vi "Test Sequence.vi"(0 "FeedBack Channel":string[](array[string])=["fgdgfvcbc", "vnfhgjkn", "21354682"], 1 "Test Name":string, 2 "Steps":T1(array[cluster]), 3 "Load":refnum<vi>) -> (6 "Emergency":bool, 7 "Out":i32, 8 "Condition":bool)   [LabVIEW 2015]
uses:
  <vilib>/Utility/error.llb/whitespace.ctl
  Galobal variable_TI.vi
  Project Setup/Globle Variable/GR_Servo.vi
panel:
  out "Wait/Poll (ms)":u32
  out "Channels (Out)":i32[](array[numeric])
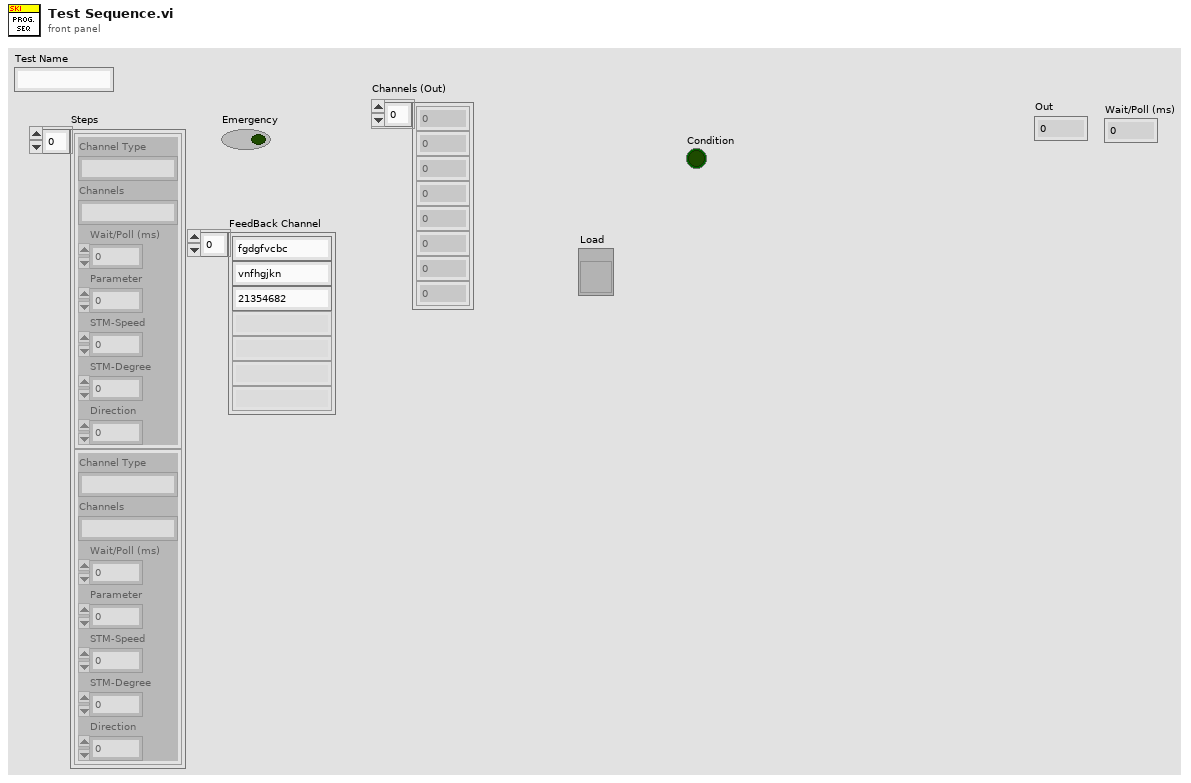
[diagram p1: front panel]
types:
  T1 = cluster{"Channel Type":string, "Channels":string, "Wait/Poll (ms)":u32, "Parameter":u8, "STM-Speed":i32, "STM-Degree":u32, "Direction":u8}[]
  T2 = cluster{"Emergency_1":bool, "Reset_2":bool, "Air Pressure_4":bool, "Safety Sensor_5":bool, "Safety Sensor_6":bool, "Barcode Rev rs_24":bool, "Clamp fwd rs_21":bool, "Servo Fault":bool, "Home _3":bool}
  T3 = cluster{"Start":bool, "Emergency ":bool, "Reset":bool, "Home":bool, "Safety":bool}
  T4 = typedef "whitespace.ctl" = u16
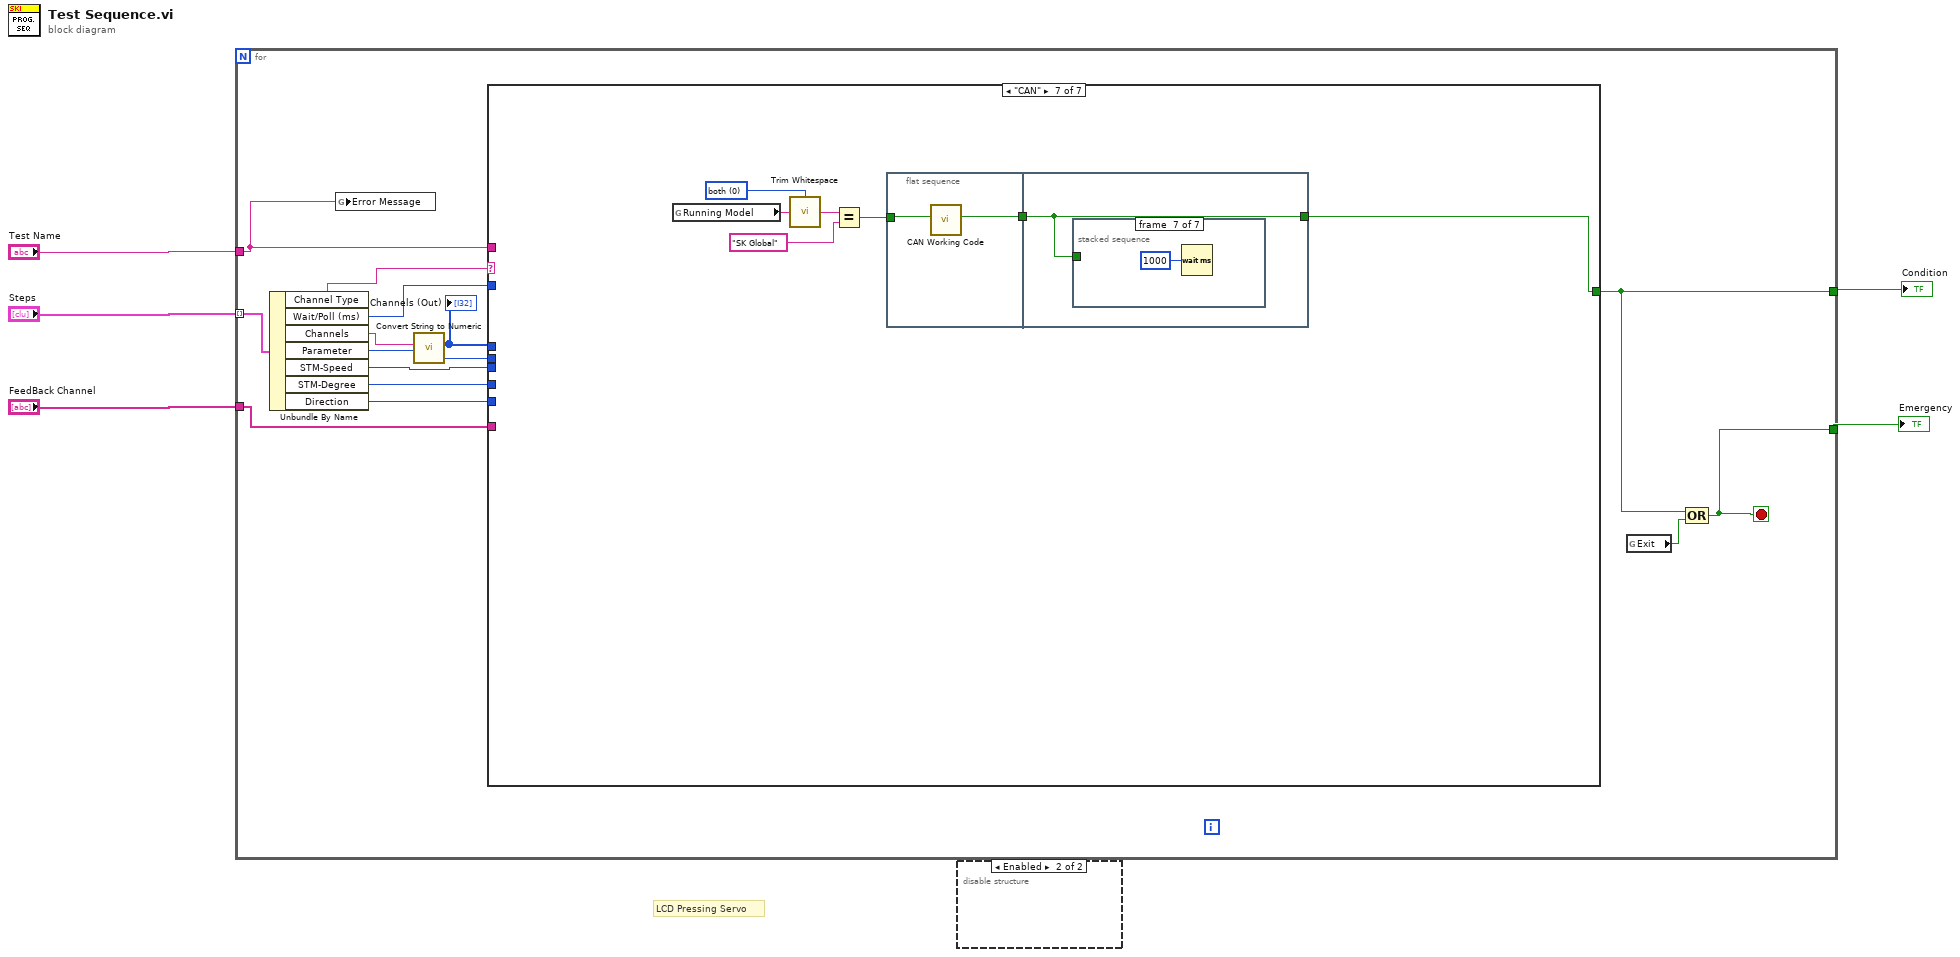
[diagram p0: block diagram]
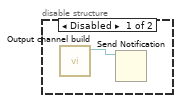
[diagram p2: hidden frame]
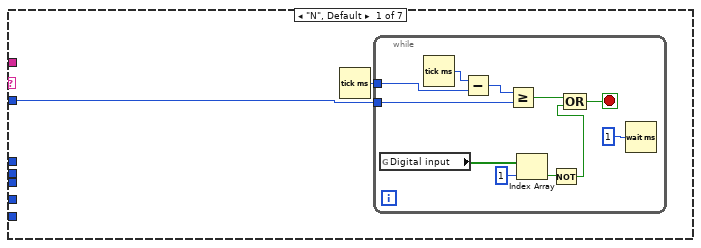
[diagram p3: hidden frame]
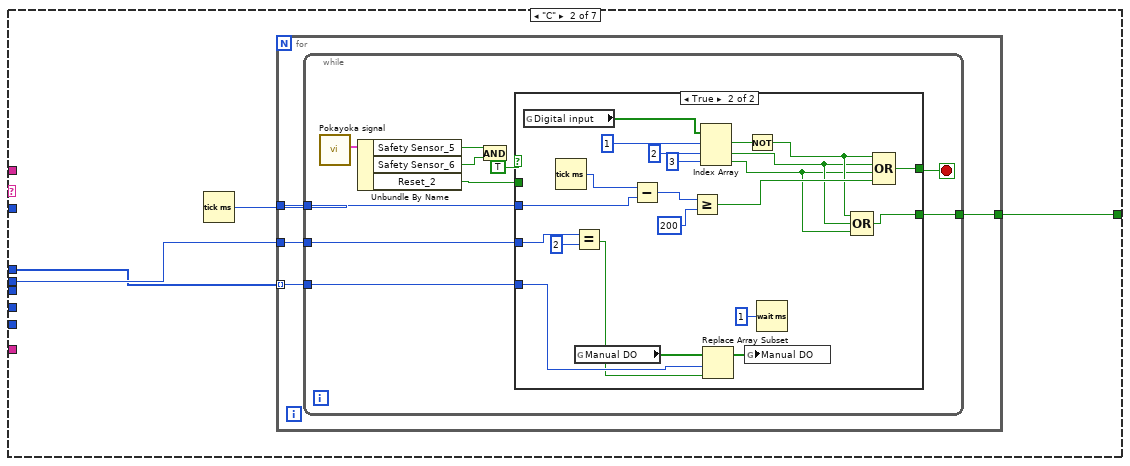
[diagram p4: hidden frame]
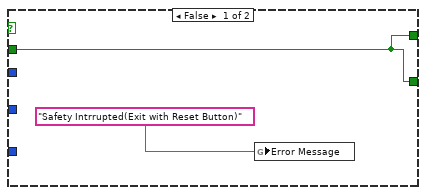
[diagram p5: hidden frame]
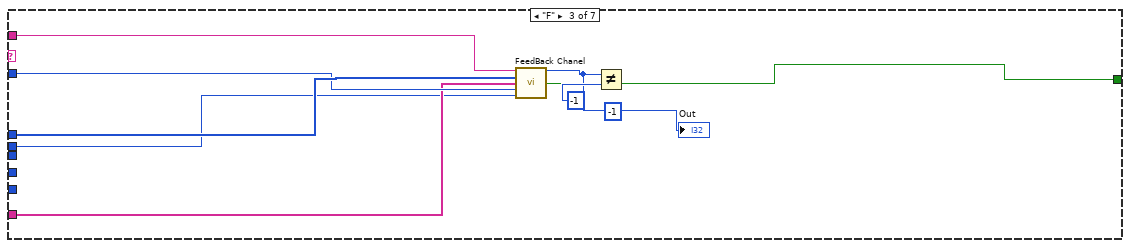
[diagram p6: hidden frame]
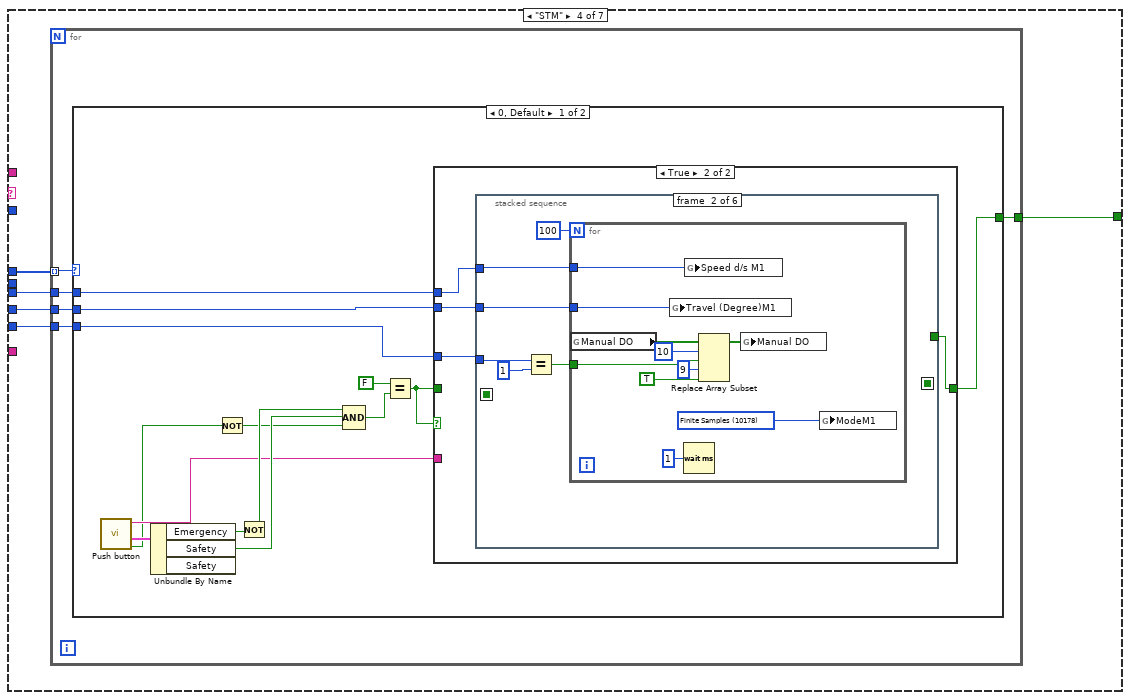
[diagram p7: hidden frame]
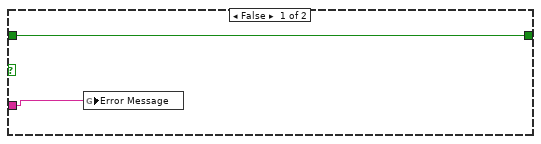
[diagram p8: hidden frame]
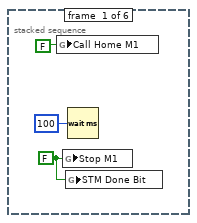
[diagram p9: hidden frame]
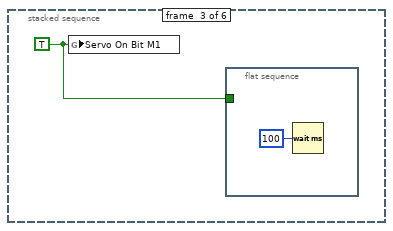
[diagram p10: hidden frame]
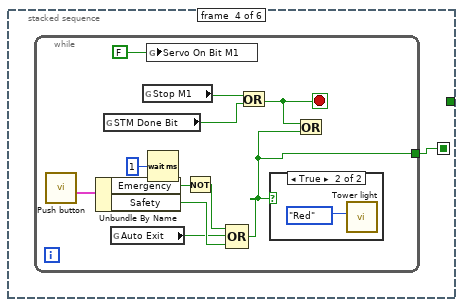
[diagram p11: hidden frame]
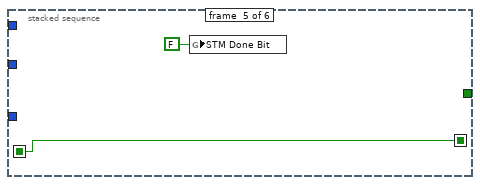
[diagram p13: hidden frame]
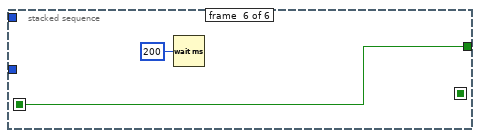
[diagram p14: hidden frame]
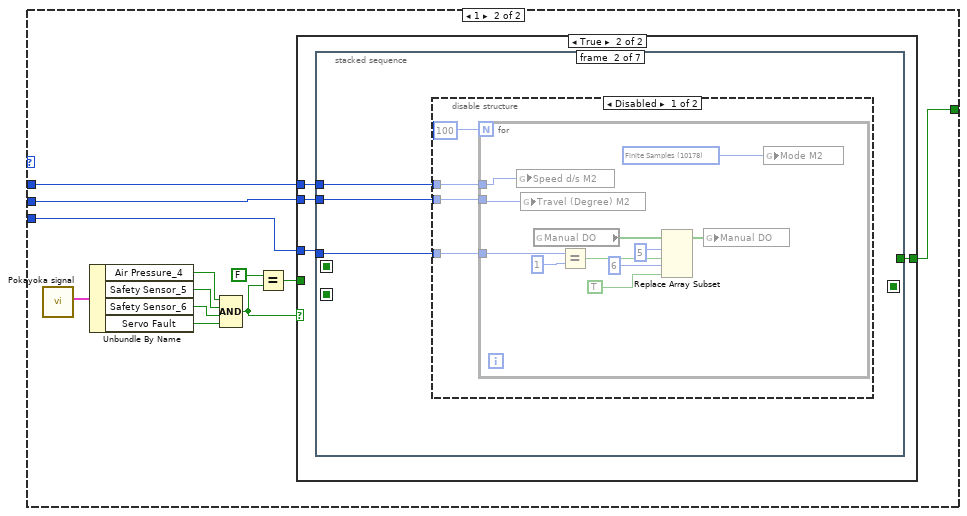
[diagram p15: hidden frame]
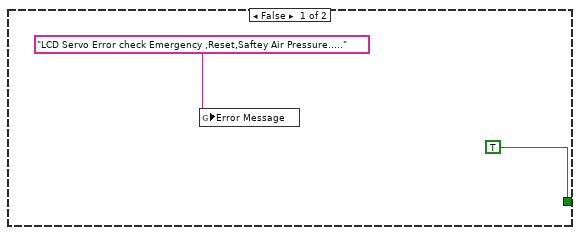
[diagram p16: hidden frame]
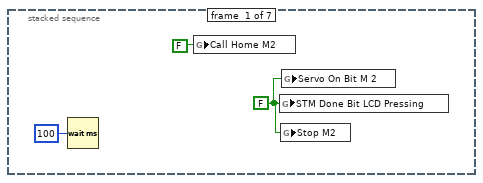
[diagram p17: hidden frame]
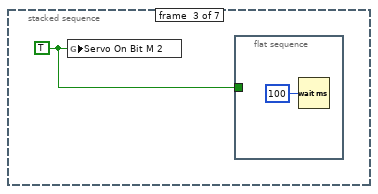
[diagram p19: hidden frame]
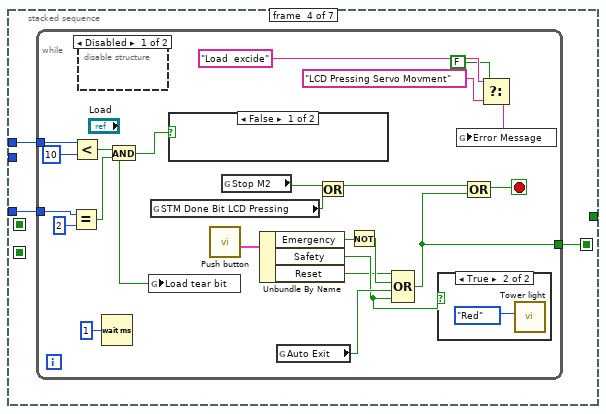
[diagram p20: hidden frame]
diagram:
  # "LCD Pressing Servo"
  n1 = for {
    tunnel: "Steps" -> [w19] mode=indexing
    tunnel: [w7] -> w5
    tunnel: "Test Name" -> [w6]
    tunnel: "FeedBack Channel" -> [w14]
    tunnel: [w12] -> w1
    stop <- w7 stop-if-true
    n2 = Unbundle By Name(w19) -> ("Channel Type"=w18:string, "Wait/Poll (ms)"=w17:u32, "Channels"=w16:string, "Parameter"=w8:u8, "STM-Speed"=w10:i32, "STM-Degree"=w9:u32, "Direction"=w11:u8)
    n3 = global write "GR_Servo.vi" "Error Message"(w6) -> ()
    n4 = call "Convert String to Numeric.vi"("Channels (A:B:C:D...) (In)"=w16) -> ("Channels (Out)"=w15:i32[])  [unwired: 9 in, 1 out]
    "Channels (Out)" <- w15
    n5 = case shown="\"CAN\"" w18 {
      tunnel: w17 -> [w20 _ w81 _ _ w273 _]
      tunnel: w15 -> [_ w34 w82 w87 w247 w274 _]
      tunnel: w11 -> [_ _ _ w86 _ _ _]
      tunnel: w6 -> [_ _ w80 _ _ _ _]
      tunnel: w14 -> [_ _ w79 _ _ _ _]
      tunnel: [_ w33 w75 w83 w245 w271 w318] -> w12
      tunnel: w10 -> [_ _ _ w85 _ _ _]
      tunnel: w9 -> [_ _ _ w84 _ _ _]
      tunnel: w8 -> [_ w36 w76 _ w246 w278 _]
      frame "N", Default {
        n6 = Tick Count (ms)() -> (millisecond timer value=w21:u32)
        n7 = while {
          tunnel: w21 -> [w31]
          tunnel: w20 -> [w26]
          stop <- w27 stop-if-true
          n8 = global read "Galobal variable_TI.vi" "Digital input"() -> (w25:bool[])
          n9 = Tick Count (ms)() -> (millisecond timer value=w32:u32)
          n10 = Subtract(x=w32, y=w31) -> (x-y=w30:u32)
          n11 = Greater Or Equal?(x=w30, y=w26) -> (x >= y?=w28:bool)
          n12 = Index Array(array=w25, index=1) -> (element=w23:bool)
          n13 = Not(x=w23) -> (.not. x?=w22:bool)
          n14 = Compound Arithmetic op=OR(w28, w22) -> (w27:bool)
          n15 = Wait (ms)(milliseconds to wait=u32 1) -> ()  [unwired: 1 out]
        }
      }
      frame "C" {
        n16 = Tick Count (ms)() -> (millisecond timer value=w35:u32)
        n17 = for {
          tunnel: w34 -> [w39] mode=indexing
          tunnel: w36 -> [w40]
          tunnel: w35 -> [w38]
          tunnel: [w37] -> w33
          n18 = while {
            tunnel: w40 -> [w50]
            tunnel: w39 -> [w49]
            tunnel: w38 -> [w48]
            tunnel: [w42] -> w37
            stop <- w43 stop-if-true
            n19 = call "Pokayoka signal.vi"() -> ("output cluster"=w47:T2)  [unwired: 10 in, 1 out]
            n20 = Unbundle By Name(w47) -> ("Safety Sensor_5"=w46:bool, "Safety Sensor_6"=w45:bool, "Reset_2"=w44:bool)
            n21 = And(x=w46, y=w45) -> ()  [unwired: 1 out]
            n22 = case shown="True" TRUE {
              tunnel: w50 -> [_ w74]
              tunnel: w49 -> [_ w73]
              tunnel: w48 -> [_ w72]
              tunnel: [w51 w71] -> w43
              tunnel: w44 -> [w51 _]
              tunnel: [w51 w53] -> w42
              frame False {
                n23 = global write "GR_Servo.vi" "Error Message"("Safety Intrrupted(Exit with Reset Button)") -> ()
              }
              frame True {
                n24 = global read "Galobal variable_TI.vi" "Digital input"() -> (w61:bool[])
                n25 = Tick Count (ms)() -> (millisecond timer value=w65:u32)
                n26 = Equal?(x=w74, y=u8 2) -> (x = y?=w66:bool)
                n27 = global read "Galobal variable_TI.vi" "Manual DO"() -> (w67:bool[])
                n28 = Subtract(x=w65, y=w72) -> (x-y=w64:u32)
                n29 = Greater Or Equal?(x=w64, y=u32 200) -> (x >= y?=w62:bool)
                n30 = Index Array(array=w61, index #1=1 ("index"), index #2=2 ("index"), index #3=3 ("index")) -> (element #1=w57:bool, element #2=w55:bool, element #3=w54:bool)
                n31 = Replace Array Subset(array=w67, new element=w66, index=w73) -> (w68:bool[])
                n32 = global write "Galobal variable_TI.vi" "Manual DO"(w68) -> ()
                n33 = Not(x=w57) -> (.not. x?=w56:bool)
                n34 = Wait (ms)(milliseconds to wait=u32 1) -> ()  [unwired: 1 out]
                n35 = Compound Arithmetic op=OR(w56, w55, w54) -> (w53:bool)
                n36 = Compound Arithmetic op=OR(w56, w55, w54, w62) -> (w71:bool)
              }
            }
          }
        }
      }
      frame "F" {
        (unwired) -1 ("Out")
        n37 = call "FeedBack Chanel.vi"("Test Name"=w80, "Channels (Int)"=w82, "FeedBack Channel"=w79, "Wait/Poll (ms)"=w81, "Parameter"=w76) -> ("Out"=w77:i32, "Fail"=w75:bool)  [unwired: 6 in, 3 out]
        "Out" <- w77
        n38 = Not Equal?(x=w77, y=-1) -> ()  [unwired: 1 out]
      }
      frame "STM" {
        n39 = for {
          tunnel: w87 -> [w92] mode=indexing
          tunnel: w86 -> [w91]
          tunnel: w85 -> [w90]
          tunnel: w84 -> [w89]
          tunnel: [w88] -> w83
          n40 = case shown="0, Default" w92 {
            tunnel: w91 -> [w104 w158]
            tunnel: w90 -> [w106 w160]
            tunnel: w89 -> [w105 w159]
            tunnel: [w101 w157] -> w88
            frame 0, Default {
              n41 = call "Push button.vi"() -> ("Air Pressure"=w95:bool, "Push Button"=w100:T3, "Error"=w96:string)  [unwired: 9 in]
              n42 = Unbundle By Name(w100) -> ("Emergency"=w99:bool, "Safety"=w97:bool)  [unwired: 1 out]
              n43 = Not(x=w95) -> (.not. x?=w93:bool)
              n44 = Not(x=w99) -> (.not. x?=w98:bool)
              n45 = Compound Arithmetic op=AND(w98, w97, w93) -> (w103:bool)
              n46 = Equal?(x=FALSE ("y"), y=w103) -> (x = y?=w94:bool)
              n47 = case shown="True" w94 {
                tunnel: w106 -> [_ w112]
                tunnel: w105 -> [_ w111]
                tunnel: w104 -> [_ w110]
                tunnel: [w108 w109] -> w101
                tunnel: w94 -> [w108 _]
                tunnel: w96 -> [w107 _]
                frame False {
                  n48 = global write "GR_Servo.vi" "Error Message"(w107) -> ()
                }
                frame True {
                  n49 = stacked-sequence {
                    seq-local: [_ _ _ w134 _ _] -> [_ _ _ _ w147 _]
                    seq-local: [_ _ _ _ w147 _] -> [_ _ _ _ _ w149]
                    tunnel: w111 -> [_ w121 _ _ _ _]
                    tunnel: w110 -> [_ w119 _ _ _ _]
                    tunnel: w112 -> [_ w117 _ _ _ _]
                    tunnel: [_ _ _ _ _ w149] -> w109
                    frame #0 {
                      w113 = FALSE ("Stop M1")
                      n50 = global write "Galobal variable_TI.vi" "Call Home M1"(FALSE ("Call Home M2")) -> ()
                      n51 = global write "Galobal variable_TI.vi" "Stop M1"(w113) -> ()
                      n52 = global write "Galobal variable_TI.vi" "STM Done Bit"(w113) -> ()
                      n53 = Wait (ms)(milliseconds to wait=u32 100) -> ()  [unwired: 1 out]
                    }
                    frame #1 {
                      n54 = Equal?(x=w119, y=u8 1) -> (x = y?=w118:bool)
                      n55 = for {
                        N: 100 -> [_]
                        tunnel: w121 -> [w131]
                        tunnel: w118 -> [w129]
                        tunnel: w117 -> [w127]
                        w130 = 10178 items=["Finite Samples"=10178, "Continuous Samples"=10123, "Hardware Timed Single Point"=12522] ("ModeM1")
                        n56 = global read "Galobal variable_TI.vi" "Manual DO"() -> (w125:bool[])
                        n57 = global write "GR_Servo.vi" "Travel (Degree)M1"(w131) -> ()
                        n58 = Wait (ms)(milliseconds to wait=u32 1) -> ()  [unwired: 1 out]
                        n59 = global write "GR_Servo.vi" "Speed d/s M1"(w127) -> ()
                        n60 = Replace Array Subset(array=w125, new element #1=w129, index #1=10 ("index"), new element #2=TRUE ("new element/subarray"), index #2=9 ("index")) -> (w128:bool[])
                        n61 = global write "Galobal variable_TI.vi" "Manual DO"(w128) -> ()
                        n62 = global write "GR_Servo.vi" "ModeM1"(w130) -> ()
                      }
                    }
                    frame #2 {
                      w132 = TRUE ("Servo On Bit")
                      n63 = global write "GR_Servo.vi" "Servo On Bit M1"(w132) -> ()
                      n64 = flat-sequence {
                        tunnel: w132 -> [_]
                        frame #0 {
                          n65 = Wait (ms)(milliseconds to wait=u32 100) -> ()  [unwired: 1 out]
                        }
                      }
                    }
                    frame #3 {
                      n66 = while {
                        tunnel: [w135] -> w134
                        stop <- w141 stop-if-true
                        n67 = call "Push button.vi"() -> ("Push Button"=w136:T3)  [unwired: 9 in, 2 out]
                        n68 = Unbundle By Name(w136) -> ("Emergency"=w137:bool, "Safety"=w140:bool)
                        n69 = global read "Galobal variable_TI.vi" "STM Done Bit"() -> (w143:bool)
                        n70 = global read "Galobal variable_TI.vi" "Auto Exit"() -> (w138:bool)
                        n71 = global read "Galobal variable_TI.vi" "Stop M1"() -> (w144:bool)
                        n72 = global write "GR_Servo.vi" "Servo On Bit M1"(FALSE ("Servo On Bit")) -> ()
                        n73 = Wait (ms)(milliseconds to wait=u32 1) -> ()  [unwired: 1 out]
                        n74 = Not(x=w137) -> (.not. x?=w139:bool)
                        n75 = Compound Arithmetic op=OR(w139, w138, w140) -> (w135:bool)
                        n76 = Or(x=w144, y=w143) -> (x .or. y?=w141:bool)
                        n77 = case shown="True" w135 {
                          frame False {
                          }
                          frame True {
                            n78 = call "Tower light.vi"("Enum"=enum16{"Green", "Red", "Yellow", "OFF"}."Red") -> ()  [unwired: 11 in]
                          }
                        }
                        n79 = Or(x=w141, y=w135) -> ()  [unwired: 1 out]
                      }
                    }
                    frame #4 {
                      n80 = global write "Galobal variable_TI.vi" "STM Done Bit"(FALSE ("STM Done Bit LCD Pressing")) -> ()
                    }
                    frame #5 {
                      n81 = Wait (ms)(milliseconds to wait=u32 200) -> ()  [unwired: 1 out]
                    }
                  }
                }
              }
            }
            frame 1 {
              n82 = call "Pokayoka signal.vi"() -> ("output cluster"=w156:T2)  [unwired: 10 in, 1 out]
              n83 = Unbundle By Name(w156) -> ("Air Pressure_4"=w155:bool, "Safety Sensor_5"=w154:bool, "Safety Sensor_6"=w153:bool, "Servo Fault"=w151:bool)
              n84 = Compound Arithmetic op=AND(w155, w154, w153, w151) -> (w152:bool)
              n85 = Equal?(x=FALSE ("y"), y=w152) -> (x = y?=w161:bool)
              n86 = case shown="True" w152 {
                tunnel: w160 -> [_ w168]
                tunnel: w159 -> [_ w167]
                tunnel: w158 -> [_ w166]
                tunnel: w161 -> [_ _]
                tunnel: [TRUE w165] -> w157
                frame False {
                  n87 = global write "GR_Servo.vi" "Error Message"("LCD Servo Error check Emergency ,Reset,Saftey Air Pressure.....") -> ()
                }
                frame True {
                  n88 = stacked-sequence {
                    seq-local: [_ _ _ w194 _ _ _] -> [_ _ _ _ w219 _ _]
                    seq-local: [_ _ _ _ w219 _ _] -> [_ _ _ _ _ w224 _]
                    seq-local: [_ _ _ _ _ w224 _] -> [_ _ _ _ _ _ w238]
                    tunnel: w167 -> [_ w174 _ _ _ _ _]
                    tunnel: w166 -> [_ w173 _ w193 _ _ w230]
                    tunnel: w168 -> [_ w172 _ w192 _ _ w231]
                    tunnel: [_ _ _ _ _ _ w236] -> w165
                    frame #0 {
                      w169 = FALSE ("STM Done Bit LCD Pressing")
                      n89 = Wait (ms)(milliseconds to wait=u32 100) -> ()  [unwired: 1 out]
                      n90 = global write "Galobal variable_TI.vi" "Call Home M2"(FALSE ("Call Home M2")) -> ()
                      n91 = global write "GR_Servo.vi" "STM Done Bit LCD Pressing"(w169) -> ()
                      n92 = global write "Galobal variable_TI.vi" "Stop M2"(w169) -> ()
                      n93 = global write "GR_Servo.vi" "Servo On Bit M 2"(w169) -> ()
                    }
                    frame #1 {
                      n94 = disable-structure shown="Disabled" {
                        disable-tunnel: w174 -> [w178 _]
                        disable-tunnel: w173 -> [w177 _]
                        disable-tunnel: w172 -> [w176 _]
                        frame Disabled {
                          n95 = for {
                            N: 100 -> [_]
                            tunnel: w178 -> [w189]
                            tunnel: w177 -> [w186]
                            tunnel: w176 -> [w183]
                            w188 = 10178 items=["Finite Samples"=10178, "Continuous Samples"=10123, "Hardware Timed Single Point"=12522] ("ModeM1")
                            n96 = global write "GR_Servo.vi" "Speed d/s M2"(w183) -> ()
                            n97 = global write "GR_Servo.vi" "Travel (Degree) M2"(w189) -> ()
                            n98 = global read "Galobal variable_TI.vi" "Manual DO"() -> (w181:bool[])
                            n99 = Equal?(x=w186, y=u8 1) -> (x = y?=w185:bool)
                            n100 = Replace Array Subset(array=w181, new element #1=w185, index #1=5 ("index"), new element #2=TRUE ("new element/subarray"), index #2=6 ("index")) -> (w184:bool[])
                            n101 = global write "Galobal variable_TI.vi" "Manual DO"(w184) -> ()
                            n102 = global write "GR_Servo.vi" "Mode M2"(w188) -> ()
                          }
                        }
                        frame Enabled {
                        }
                      }
                    }
                    frame #2 {
                      w190 = TRUE ("Servo On Bit")
                      n103 = global write "GR_Servo.vi" "Servo On Bit M 2"(w190) -> ()
                      n104 = flat-sequence {
                        tunnel: w190 -> [_]
                        frame #0 {
                          n105 = Wait (ms)(milliseconds to wait=u32 100) -> ()  [unwired: 1 out]
                        }
                      }
                    }
                    frame #3 {
                      n106 = while {
                        tunnel: [w208] -> w194
                        tunnel: w193 -> [w203]
                        tunnel: w192 -> [w201]
                        stop <- w209 stop-if-true
                        n107 = Equal?(x=w203, y=u8 2) -> (x = y?=w198:bool)
                        n108 = Less?(x=w201, y=10) -> (x < y?=w199:bool)
                        n109 = disable-structure shown="Disabled" {
                          frame Disabled {
                          }
                          frame Enabled {
                          }
                        }
                        n110 = Wait (ms)(milliseconds to wait=u32 1) -> ()  [unwired: 1 out]
                        n111 = And(x=w199, y=w198) -> (x .and. y?=w196:bool)
                        n112 = global write "Galobal variable_TI.vi" "Load tear bit"(w196) -> ()
                        n113 = global read "GR_Servo.vi" "STM Done Bit LCD Pressing"() -> (w215:bool)
                        n114 = case shown="False" w196 {
                          frame False {
                          }
                          frame True {
                          }
                        }
                        n115 = call "Push button.vi"() -> ("Push Button"=w214:T3)  [unwired: 9 in, 2 out]
                        n116 = global read "Galobal variable_TI.vi" "Stop M2"() -> (w216:bool)
                        n117 = Unbundle By Name(w214) -> ("Emergency"=w213:bool, "Safety"=w207:bool, "Reset"=w195:bool)
                        n118 = global read "Galobal variable_TI.vi" "Auto Exit"() -> (w212:bool)
                        n119 = Or(x=w216, y=w215) -> (x .or. y?=w210:bool)
                        n120 = Not(x=w213) -> (.not. x?=w211:bool)
                        n121 = Compound Arithmetic op=OR(w195, w211, w212, w207) -> (w208:bool)
                        n122 = case shown="True" w207 {
                          frame False {
                          }
                          frame True {
                            n123 = call "Tower light.vi"("Enum"=enum16{"Green", "Red", "Yellow", "OFF"}."Red") -> ()  [unwired: 11 in]
                          }
                        }
                        n124 = Compound Arithmetic op=OR(w210, w208) -> (w209:bool)
                        n125 = Select(t="Load  excide", s=FALSE, f="LCD Pressing Servo Movment") -> (s? t:f=w204:string)
                        n126 = global write "GR_Servo.vi" "Error Message"(w204) -> ()
                      }
                    }
                    frame #4 {
                      (unwired) FALSE
                      n127 = Wait (ms)(milliseconds to wait=u32 1) -> ()  [unwired: 1 out]
                      n128 = global write "GR_Servo.vi" "Servo On Bit M 2"(FALSE ("Servo On Bit")) -> ()
                      n129 = global write "GR_Servo.vi" "STM Done Bit LCD Pressing"(FALSE ("STM Done Bit LCD Pressing")) -> ()
                    }
                    frame #5 {
                      n130 = disable-structure shown="Disabled" {
                        frame Disabled {
                          n131 = local read "Load"() -> (w226:refnum<vi>)
                          n132 = call "Load Value.vi"("String in"=w226) -> (1:w227, "Load Cell"=w228:dbl)  [unwired: 9 in]
                          n133 = Greater?(x=w228, y=w227) -> ()  [unwired: 1 out]
                        }
                        frame Enabled {
                        }
                      }
                      n134 = Wait (ms)(milliseconds to wait=u32 100) -> ()  [unwired: 1 out]
                      n135 = global write "Galobal variable_TI.vi" "Load tear bit"(FALSE ("Load tear bit")) -> ()
                    }
                    frame #6 {
                      n136 = Equal?(x=w230, y=u8 2) -> (x = y?=w235:bool)
                      n137 = Less?(x=w231, y=10) -> (x < y?=w234:bool)
                      n138 = And(x=w234, y=w235) -> ()  [unwired: 1 out]
                      n139 = case shown="True" FALSE {
                        tunnel: [FALSE w242] -> w237
                        frame False {
                        }
                        frame True {
                          n140 = global read "Galobal variable_TI.vi" "Load Status"() -> (w243:string)
                          n141 = global write "GR_Servo.vi" "Error Color"(1 ("Error Color")) -> ()
                          n142 = Equal?(x=w243, y="Fail") -> (x = y?=w242:bool)
                          n143 = global write "GR_Servo.vi" "Error Message"("Load NG" ("Error Message")) -> ()
                        }
                      }
                      n144 = Or(x=w238, y=w237) -> (x .or. y?=w236:bool)
                    }
                  }
                }
              }
            }
          }
        }
      }
      frame "CAM" {
        n145 = for {
          tunnel: w247 -> [w250] mode=indexing
          tunnel: w246 -> [w249]
          tunnel: [w248] -> w245
          n146 = case shown="0, Default" w250 {
            tunnel: w249 -> [_ _]
            tunnel: [w251 _] -> w248
            frame 0, Default {
              n147 = stacked-sequence {
                seq-local: [w252 _] -> [_ w269]
                tunnel: [_ w269] -> w251
                frame #0 {
                  n148 = while {
                    tunnel: [w261] -> w252
                    stop <- w263 stop-if-true
                    n149 = global read "Galobal variable_TI.vi" "Digital input"() -> (w257:bool[])
                    n150 = call "Push button.vi"() -> ("Push Button"=w267:T3)  [unwired: 9 in, 2 out]
                    n151 = global read "Galobal variable_TI.vi" "Camera Result"() -> (w259:string)
                    n152 = Unbundle By Name(w267) -> ("Emergency"=w266:bool, "Reset"=w264:bool)
                    n153 = Index Array(array=w257, index #1=12 ("index"), index #2=13 ("index")) -> (element #1=w253:bool, element #2=w254:bool)
                    n154 = Equal?(x=w259, y="2") -> ()  [unwired: 1 out]
                    n155 = Equal?(x=w259, y="1") -> ()  [unwired: 1 out]
                    n156 = Not(x=w266) -> (.not. x?=w265:bool)
                    n157 = Compound Arithmetic op=OR(w265, w264, w254) -> (w261:bool)
                    n158 = Wait (ms)(milliseconds to wait=u32 1) -> ()  [unwired: 1 out]
                    n159 = Compound Arithmetic op=OR(w261, w253) -> (w263:bool)
                  }
                }
                frame #1 {
                  n160 = global write "Galobal variable_TI.vi" "Camera Result"("" ("Camera Result")) -> ()
                }
              }
            }
            frame 1 {
              # "LCD Pressing Servo"
            }
          }
        }
      }
      frame "BAR" {
        # "0- Mic Code Read\n1-dail gauge lh\n2-dail gauge RH\n3-dail Strip up\n4-dail strip dn"
        n161 = Equal?(x=w278, y=u8 2) -> (x = y?=w276:bool)
        n162 = Index Array(array=w274) -> (element=w272:i32)  [unwired: 1 in]
        n163 = case shown="0, Default" w272 {
          tunnel: w276 -> [w285 w302 w307 w311 w314]
          tunnel: [w281 w301 w306 w310 w315] -> w275
          tunnel: [w279 FALSE ("Fail") FALSE ("Fail") FALSE ("Fail") FALSE ("Fail")] -> w270
          frame 0, Default {
            n164 = case shown="True" w285 {
              tunnel: [FALSE ("exit") w299] -> w281
              tunnel: [_ w298] -> w283
              frame False {
              }
              frame True {
                n165 = call "Barcode read.vi"() -> ("exit"=w299:bool, "Barcode Scan Bit"=w298:bool)  [unwired: 7 in, 3 out]
              }
            }
            n166 = global read "Galobal variable_TI.vi" "Tracbility"() -> (w284:bool)
            n167 = Not(x=w281) -> (.not. x?=w280:bool)
            n168 = And(x=w280, y=w284) -> (x .and. y?=w282:bool)
            n169 = case shown="True" w282 {
              tunnel: w283 -> [_ w290]
              tunnel: [FALSE ("Fail") w289] -> w279
              frame False {
              }
              frame True {
                n170 = flat-sequence {
                  tunnel: w290 -> [w292]
                  tunnel: [w292] -> w287
                  tunnel: [w294] -> w288
                  tunnel: w287 -> [w294]
                  tunnel: [w295] -> w289
                  tunnel: w288 -> [w296]
                  frame #0 {
                    n171 = global write "Galobal variable_TI.vi" "RPT Read"(TRUE ("RPT Read")) -> ()
                  }
                  frame #1 {
                    n172 = Wait (ms)(milliseconds to wait=u32 500) -> ()  [unwired: 1 out]
                  }
                  frame #2 {
                    n173 = call "RPT Comaristion.vi"("True"=w296) -> ("Fail"=w295:bool)  [unwired: 10 in]
                  }
                }
              }
            }
          }
          frame 1 {
            n174 = case shown="True" w302 {
              tunnel: [FALSE ("exit") w304] -> w301
              frame False {
              }
              frame True {
                n175 = call "Dail LH_Barcode read.vi"() -> ("exit"=w304:bool)  [unwired: 8 in, 3 out]
              }
            }
          }
          frame 2 {
            n176 = case shown="True" w307 {
              tunnel: [_ w308] -> w306
              frame False {
              }
              frame True {
                n177 = call "Dail RH_Barcode read.vi"() -> ("exit"=w308:bool)  [unwired: 8 in, 3 out]
              }
            }
          }
          frame 3 {
            n178 = case shown="True" w311 {
              tunnel: [_ w312] -> w310
              frame False {
              }
              frame True {
                n179 = call "Dail Strip Up_Barcode read.vi"() -> ("exit"=w312:bool)  [unwired: 8 in, 3 out]
              }
            }
          }
          frame 4 {
            n180 = case shown="True" w314 {
              tunnel: [_ w316] -> w315
              frame False {
              }
              frame True {
                n181 = call "Dail Strip Dn_Barcode read.vi"() -> ("exit"=w316:bool)  [unwired: 8 in, 3 out]
              }
            }
          }
        }
        n182 = Or(x=w270, y=w275) -> (x .or. y?=w271:bool)
        "Wait/Poll (ms)" <- w273
      }
      frame "CAN" {
        w322 = T4 0 items=["both", "start of string", "end of string"] ("location (both)")
        n183 = global read "Galobal variable_TI.vi" "Running Model"() -> (w321:string)
        n184 = call <vilib>:"Trim Whitespace.vi"("string"=w321, "location (both)"=w322) -> ("trimmed string"=w320:string)
        n185 = Equal?(x=w320, y="SK Global") -> (x = y?=w319:bool)
        n186 = flat-sequence {
          tunnel: w319 -> [w325]
          tunnel: [w324] -> w317
          tunnel: [w326] -> w318
          tunnel: w317 -> [w326]
          frame #0 {
            n187 = call "CAN Working Code.vi"("G(T) SK&VW(F)"=w325) -> ("Fail"=w324:bool)  [unwired: 10 in]
          }
          frame #1 {
            n188 = stacked-sequence {
              tunnel: w326 -> [_ _ _ _ _ _ _]
              frame #0 {
                n189 = global write "Galobal variable_TI.vi" "CAM Trigger Right"(FALSE ("CAM Trigger Left")) -> ()
              }
              frame #1 {
                n190 = Wait (ms)(milliseconds to wait=u32 250) -> ()  [unwired: 1 out]
              }
              frame #2 {
                n191 = global write "Galobal variable_TI.vi" "CAM Trigger Left"(FALSE ("CAM Trigger Right")) -> ()
              }
              frame #3 {
                n192 = Wait (ms)(milliseconds to wait=u32 250) -> ()  [unwired: 1 out]
              }
              frame #4 {
                n193 = global write "Galobal variable_TI.vi" "CAM Trigger Center"(FALSE ("CAM Trigger Center")) -> ()
              }
              frame #5 {
                n194 = Wait (ms)(milliseconds to wait=u32 250) -> ()  [unwired: 1 out]
              }
              frame #6 {
                n195 = Wait (ms)(milliseconds to wait=u32 1000) -> ()  [unwired: 1 out]
              }
            }
          }
        }
      }
    }
    n196 = global read "Galobal variable_TI.vi" "Exit"() -> (w13:bool)
    n197 = Compound Arithmetic op=OR(w12, w13) -> (w7:bool)
  }
  "Emergency" <- w5
  "Condition" <- w1
  n198 = disable-structure shown="Enabled" {
    frame Disabled {
      n199 = call "Output channel build.vi"() -> ("Output channel"=w334:refnum<notifier>)  [unwired: 11 in]
      n200 = Send Notification(notifier=w334) -> ()  [unwired: 2 in, 2 out]
    }
    frame Enabled {
    }
  }
